vi "Input1.vi"(0 "Current * 10^input":dbl, 4 "Scopez":dbl, 5 "Drag":dbl, 6 "FH":dbl, 7 "Signal in":dbl, 8 "FW":dbl, 9 "Scopex":dbl, 10 "Z origin":dbl, 11 "X origin":dbl) -> (1 "Scaled Current":dbl)   [LabVIEW 2019]
uses:
  Program Files/National Instruments/LabVIEW 2019/user.lib/HapticSTM/HapticSTM.lvlib
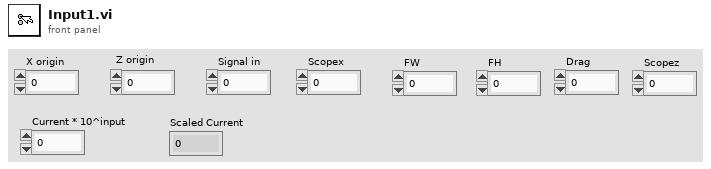
[diagram p1: front panel]
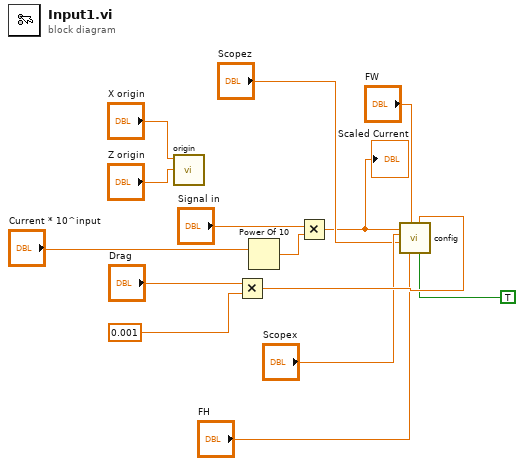
[diagram p0: block diagram]
diagram:
  n1 = call "origin.vi"("zorg"="Z origin", "xorg"="X origin") -> ()  [unwired: 10 in]
  n2 = Multiply(x="Drag", y=0.001) -> (x*y=w10:dbl)
  n3 = Power Of 10(x="Current * 10^input") -> (10^x=w4:dbl)
  n4 = Multiply(x="Signal in", y=w4) -> (x*y=w2:dbl)
  "Scaled Current" <- w2
  n5 = call "config.vi"("feedback"=TRUE, "dragc"=w10, "sizeofimgz"="FH", "sizeofimgx"="FW", "scopez"="Scopez", "scopex"="Scopex", "ypos"=w2) -> ()  [unwired: 5 in]
